vi "Save config.vi"(8 "error in (no error)":errorcluster, 11 "Arduino config":T1) -> (0 "error out":errorcluster)   [LabVIEW 2020]
uses:
  controls/Arduino config.ctl
  <vilib>/Utility/config.llb/Write Key (String).vi
  <vilib>/Utility/config.llb/NI_LVConfig.lvlib
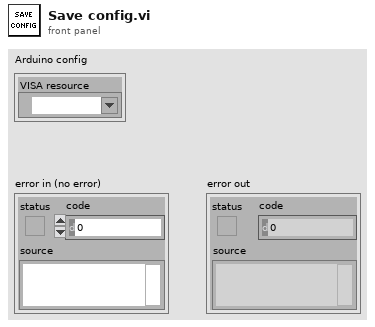
[diagram p1: front panel]
types:
  T1 = typedef "Arduino config.ctl" = cluster{"VISA resource":refnum<visa-resource-name>}
  T2 = typedef "NI_LVConfig.lvlib/Config Data RefNum.ctl" = refnum<k1>
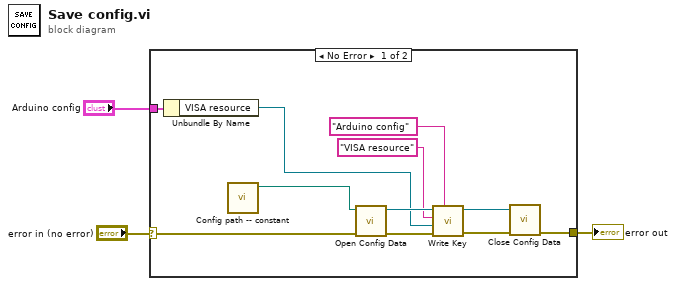
[diagram p0: block diagram]
diagram:
  n1 = case shown="No Error" "error in (no error)" {
    selector: "error in (no error)" -> [w13 w15]
    tunnel: [w10 w15] -> w2
    tunnel: "Arduino config" -> [w6 _]
    frame No Error {
      n2 = Unbundle By Name(w6) -> ("VISA resource"=w4:refnum<visa-resource-name>)
      n3 = call "Config path -- constant.vi"() -> ("appended path"=w14:path)  [unwired: 11 in]
      n4 = call <vilib>:"Open Config Data.vi"("error in (no error)"=w13, "configuration file path"=w14) -> ("error out"=w12:errorcluster, "refnum"=w8:T2)  [unwired: 7 in, 1 out]
      n5 = call-poly <vilib>:"Write Key.vi"("section"="Arduino config", "error in (no error)"=w12, "value"=w4, "key"="VISA resource", "refnum"=w8) -> ("error out"=w11:errorcluster, "refnum out"=w7:T2)  [unwired: 4 in, 1 out]
      n6 = call <vilib>:"Close Config Data.vi"("error in (no error)"=w11, "refnum"=w7) -> ("error out"=w10:errorcluster)  [unwired: 8 in, 1 out]
    }
    frame Error {
    }
  }
  "error out" <- w2
